vi "DataAcquisition.vi"() -> ()   [LabVIEW 2013]
uses:
  GlobleVar/SamplingRate.vi
  GlobleVar/stack_size.vi
  GlobleVar/Data.vi
  <vilib>/DAQmx/create/channels.llb/DAQmx Create Channel (AI-Voltage-Basic).vi
  <vilib>/DAQmx/configure/timing.llb/DAQmx Timing (Sample Clock).vi
  GlobleVar/segment_size.vi
  <vilib>/DAQmx/read.llb/DAQmx Read (Analog 2D DBL NChan NSamp).vi
panel:
  out "Waveform Graph":dbl[][](graph)
  out "Data":dbl[][](array[numeric])
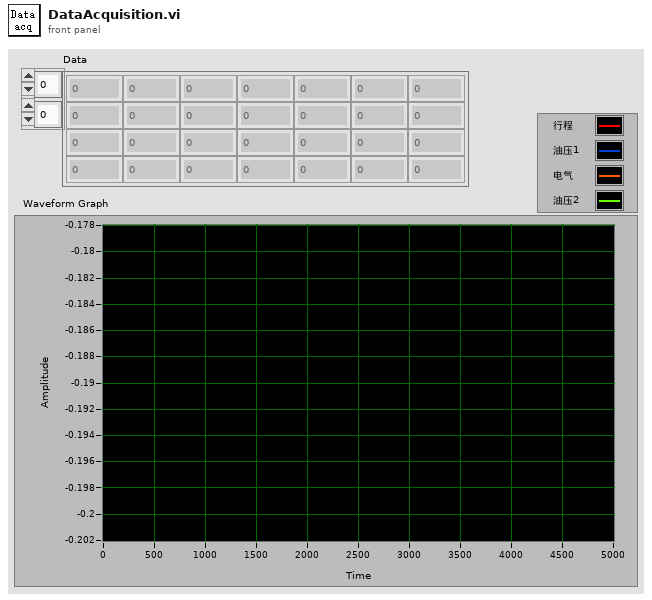
[diagram p1: front panel]
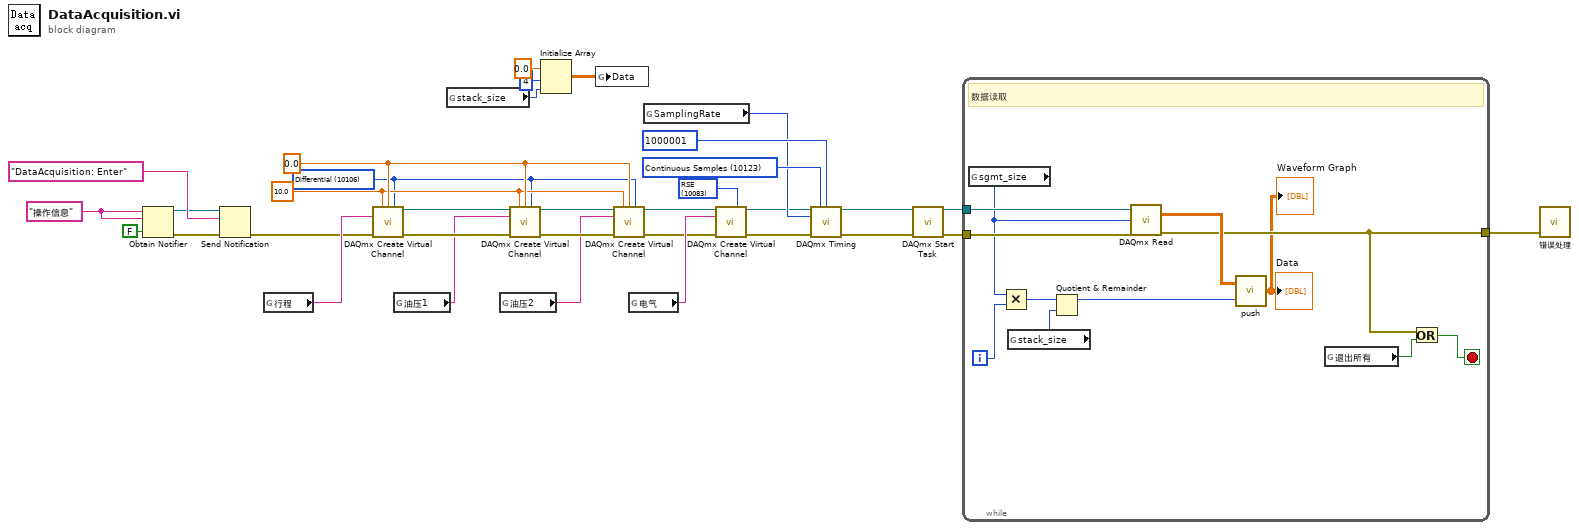
[diagram p0: block diagram]
diagram:
  w1 = 10083 items=["default"=-1, "RSE"=10083, "NRSE"=10078, "Differential"=10106, "Pseudodifferential"=12529] ("input terminal configuration")
  w2 = 10106 items=["default"=-1, "RSE"=10083, "NRSE"=10078, "Differential"=10106, "Pseudodifferential"=12529] ("input terminal configuration")
  w7 = "操作信息"
  w30 = 0.0 ("minimum value")
  w29 = 10.0 ("maximum value")
  w32 = 10123 items=["Finite Samples"=10178, "Continuous Samples"=10123, "Hardware Timed Single Point"=12522] ("sample mode")
  n1 = Obtain Notifier(name (unnamed)=w7, notification data type=w7, create if not found? (T)=FALSE) -> (notifier out=w5:refnum<notifier>, error out=w4:errorcluster)  [unwired: 1 in, 1 out]
  n2 = Send Notification(notification="DataAcquisition: Enter" ("string/path"), notifier=w5, error in (no error)=w4) -> (error out=w3:errorcluster)  [unwired: 1 out]
  n3 = global read "AI端口_行程.vi" "行程"() -> (w25:tag)
  n4 = call-poly <vilib>:"DAQmx Create Virtual Channel.vi"("maximum value"=w29, "minimum value"=w30, "input terminal configuration"=w2, "physical channels"=w25, "error in"=w3) -> ("task out"=w31:refnum<k21>, "error out"=w27:errorcluster)  [unwired: 9 in]
  n5 = global read "AI端口_油压1.vi" "油压1"() -> (w24:tag)
  n6 = global read "stack_size.vi" "stack_size"() -> (w14:i32)
  n7 = global read "AI端口_油压2.vi" "油压2"() -> (w23:tag)
  n8 = call-poly <vilib>:"DAQmx Create Virtual Channel.vi"("task in"=w31, "maximum value"=w29, "minimum value"=w30, "input terminal configuration"=w2, "physical channels"=w24, "error in"=w27) -> ("task out"=w28:refnum<k21>, "error out"=w26:errorcluster)  [unwired: 8 in]
  n9 = Initialize Array(0.0 ("element"), 4 ("dimension size"), w14) -> (w17:dbl[][])
  n10 = global write "Data.vi" "Data"(w17) -> ()
  n11 = call-poly <vilib>:"DAQmx Create Virtual Channel.vi"("task in"=w28, "maximum value"=w29, "minimum value"=w30, "input terminal configuration"=w2, "physical channels"=w23, "error in"=w26) -> ("task out"=w12:refnum<k21>, "error out"=w9:errorcluster)  [unwired: 8 in]
  n12 = global read "AI端口_电气.vi" "电气"() -> (w13:tag)
  n13 = global read "SamplingRate.vi" "SamplingRate"() -> (w19:i32)
  n14 = call-poly <vilib>:"DAQmx Create Virtual Channel.vi"("task in"=w12, "input terminal configuration"=w1, "physical channels"=w13, "error in"=w9) -> ("task out"=w11:refnum<k21>, "error out"=w10:errorcluster)  [unwired: 10 in]
  n15 = call-poly <vilib>:"DAQmx Timing.vi"("task/channels in"=w11, "sample mode"=w32, "samples per channel"=1000001, "rate"=w19, "error in"=w10) -> ("task out"=w34:refnum<k21>, "error out"=w33:errorcluster)  [unwired: 9 in]
  n16 = call <vilib>:"DAQmx Start Task.vi"("task/channels in"=w34, "error in"=w33) -> ("task out"=w22:refnum<k21>, "error out"=w21:errorcluster)  [unwired: 12 in]
  n17 = while {
    tunnel: w22 -> [w46]
    tunnel: w21 -> [w45]
    tunnel: [w41] -> w18
    i -> [w39]
    stop <- w42 stop-if-true
    # "数据读取"
    n18 = global read "segment_size.vi" "sgmt_size"() -> (w40:i32)
    n19 = Multiply(x=w40, y=w39) -> (x*y=w38:i32)
    n20 = global read "stack_size.vi" "stack_size"() -> (w37:i32)
    n21 = Quotient & Remainder(x=w38, y=w37) -> (x-y*floor(x/y)=w36:i32)  [unwired: 1 out]
    n22 = call-poly <vilib>:"DAQmx Read.vi"("task/channels in"=w46, "number of samples per channel"=w40, "error in"=w45) -> ("data"=w44:dbl[][], "error out"=w41:errorcluster)  [unwired: 10 in, 1 out]
    n23 = call "push.vi"("ptr_write"=w36, "Data in"=w44) -> ("Data"=→"Data" →"Waveform Graph":dbl[][])
    n24 = global read "退出所有.vi" "退出所有"() -> (w43:bool)
    n25 = Or(x=w41, y=w43) -> (x .or. y?=w42:bool)
  }
  n26 = call "错误处理.vi"("error in (no error)"=w18) -> ()  [unwired: 2 in]
